vi "Textbox.vi"(7 "Message":string, 8 "error in (no error)":errorcluster, 9 "Textbox Location":T1, 10 "Textbox Name":string, 11 "ITX Commands in":refnum<class "ITX Commands.lvclass">) -> (0 "error out":errorcluster, 3 "ITX Commands out":refnum<class "ITX Commands.lvclass">)   [LabVIEW 2019, in "ITX Commands.lvclass"]
uses:
  ITX Commands.lvclass
  ITX Commands.lvclass/ITX Commands.ctl
panel:
  out "resulting string":string
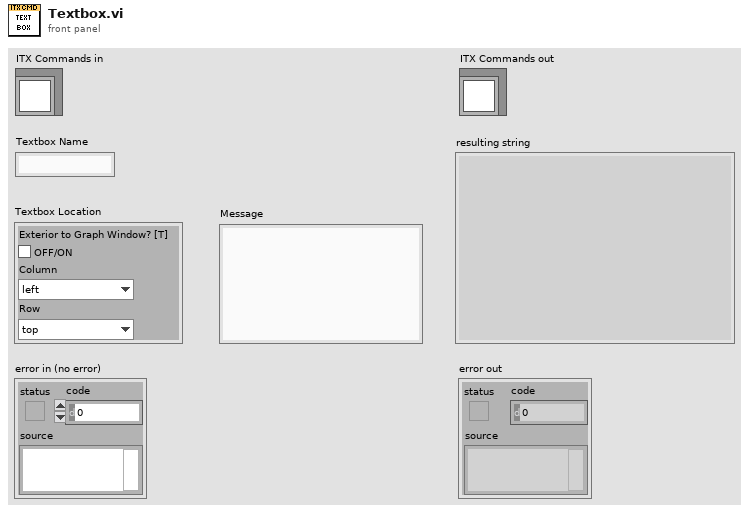
[diagram p1: front panel]
types:
  T1 = cluster{"Exterior to Graph Window? [T]":bool, "Column":enum16{"left", "middle", "right"}, "Row":enum16{"top", "center", "bottom"}}
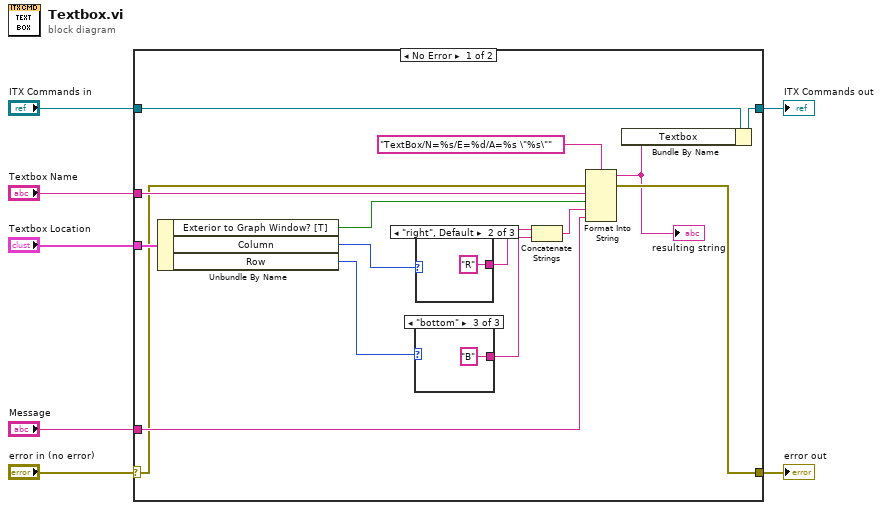
[diagram p0: block diagram]
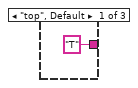
[diagram p2: hidden frame]
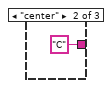
[diagram p3: hidden frame]
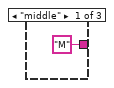
[diagram p4: hidden frame]
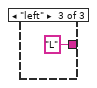
[diagram p5: hidden frame]
diagram:
  n1 = case shown="No Error" "error in (no error)" {
    selector: "error in (no error)" -> [w12 w30]
    tunnel: [w11 w30] -> w6
    tunnel: [w10 w29] -> w4
    tunnel: "ITX Commands in" -> [w22 w29]
    tunnel: "Textbox Location" -> [w16 _]
    tunnel: "Textbox Name" -> [w15 _]
    tunnel: "Message" -> [w14 _]
    frame No Error {
      n2 = Unbundle By Name(w16) -> ("Exterior to Graph Window? [T]"=w8:bool, "Column"=w20:enum16{"left", "middle", "right"}, "Row"=w13:enum16{"top", "center", "bottom"})
      n3 = case shown="\"bottom\"" w13 {
        tunnel: ["T" "C" "B"] -> w18
        frame "top", Default {
        }
        frame "center" {
        }
        frame "bottom" {
        }
      }
      n4 = case shown="\"right\", Default" w20 {
        tunnel: ["M" "R" "L"] -> w19
        frame "middle" {
        }
        frame "right", Default {
        }
        frame "left" {
        }
      }
      n5 = Concatenate Strings(w19, w18) -> (w17:string)
      n6 = Format Into String(format string="TextBox/N=%s/E=%d/A=%s \"%s\"", error in=w12, w15, w8, w17, w14) -> (resulting string=w9:string, error out=w11:errorcluster)  [unwired: 1 in]
      "resulting string" <- w9
      n7 = Bundle By Name(cluster=w22, "Textbox"=w9) -> (w10:refnum<class "ITX Commands.lvclass">)
    }
    frame Error {
    }
  }
  "error out" <- w6
  "ITX Commands out" <- w4
